vi "Andor_iXon_GetData.vi"(8 "error in":errorcluster, 11 "input cluster":T6) -> (0 "error out":errorcluster, 2 "Array 3":i32[][][](array[numeric]), 3 "array":i32[](array[numeric]))   [LabVIEW 2009]
uses:
  atmcd32d.llb/AcquisitionMode_mode typedef.ctl
  atmcd32d.llb/ReadMode_mode typedef.ctl
  atmcd32d.llb/TriggerMode_mode typedef.ctl
  atmcd32d.llb/Shutter_type typedef.ctl
  atmcd32d.llb/Shutter_mode typedef.ctl
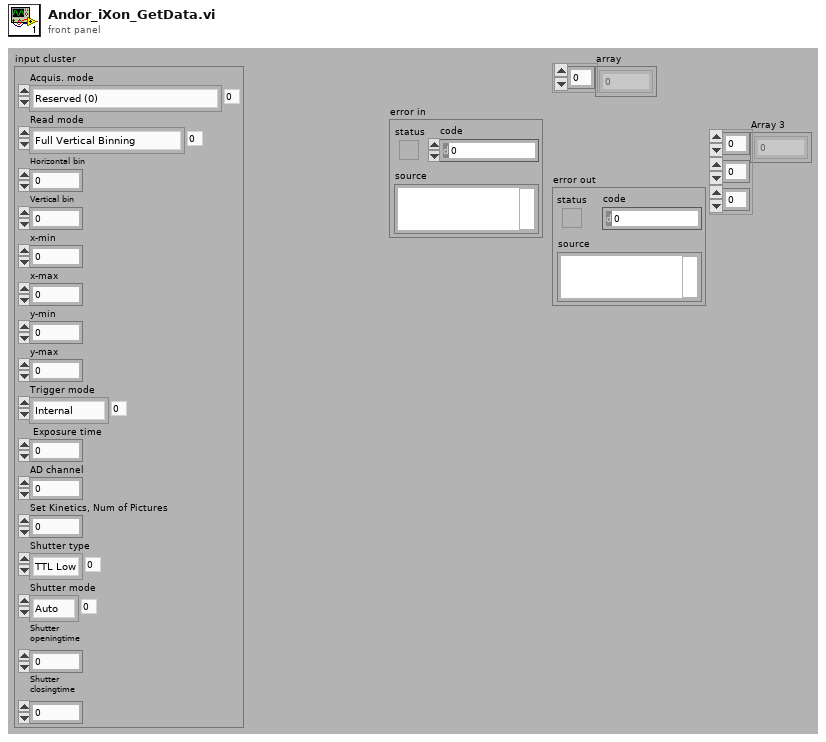
[diagram p1: front panel]
types:
  T1 = typedef "AcquisitionMode_mode typedef.ctl" = enum16{"Reserved (0)", "Single Scan", "Accumulate", "Kinetics", "Fast Kinetics", "Run Till Abort", "Reserved (6)", "Reserved (7)", "Reserved (8)", "Time Delayed Integration"}
  T2 = typedef "ReadMode_mode typedef.ctl" = enum16{"Full Vertical Binning", "Multi-Track", "Random-Track", "Single-Track", "Image"}
  T3 = typedef "TriggerMode_mode typedef.ctl" = enum16{"Internal", "External", "N/A (2)", "N/A (3)", "N/A (4)", "N/A (5)", "External Start"}
  T4 = typedef "Shutter_type typedef.ctl" = enum16{"TTL Low", "TTL High"}
  T5 = typedef "Shutter_mode typedef.ctl" = enum16{"Auto", "Open", "Close"}
  T6 = cluster{"Acquis. mode":T1, "Read mode":T2, "Horizontal bin":i32, "Vertical bin":i32, "x-min":i32, "x-max":i32, "y-min":i32, "y-max":i32, "Trigger mode":T3, " Exposure time":sgl, "AD channel":i32, "Set Kinetics, Num of Pictures":i32, "Shutter type":T4, "Shutter mode":T5, "Shutter\nopeningtime":i32, "Shutter\nclosingtime":i32}
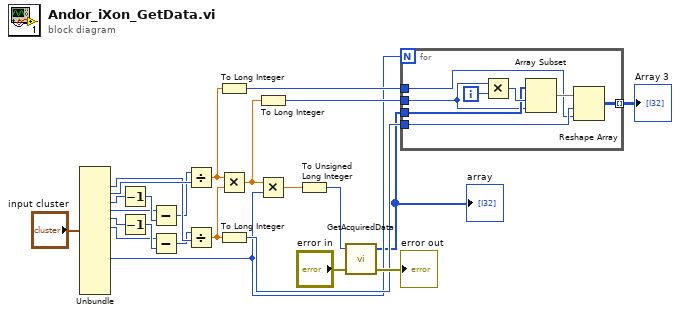
[diagram p0: block diagram]
diagram:
  n1 = Unbundle("input cluster") -> ("Horizontal bin"=w20:i32, "Vertical bin"=w21:i32, "x-min"=w11:i32, "x-max"=w4:i32, "y-min"=w3:i32, "y-max"=w5:i32, "Set Kinetics, Num of Pictures"=w14:i32)  [unwired: 9 out]
  n2 = Decrement(x=w11) -> (x-1=w10:i32)
  n3 = Decrement(x=w3) -> (x-1=w9:i32)
  n4 = Subtract(x=w4, y=w10) -> (x-y=w13:i32)
  n5 = Subtract(x=w5, y=w9) -> (x-y=w12:i32)
  n6 = Divide(x=w13, y=w21) -> (x/y=w7:dbl)
  n7 = Divide(x=w12, y=w20) -> (x/y=w8:dbl)
  n8 = To Long Integer(number=w7) -> (32bit integer=w19:i32)
  n9 = Multiply(x=w7, y=w8) -> (x*y=w15:dbl)
  n10 = To Long Integer(number=w8) -> (32bit integer=w18:i32)
  n11 = To Long Integer(number=w15) -> (32bit integer=w16:i32)
  n12 = Multiply(x=w15, y=w14) -> (x*y=w22:dbl)
  n13 = To Unsigned Long Integer(number=w22) -> (unsigned 32bit integer=w1:u32)
  n14 = call "GetAcquiredData.vi"("error in (no error)"="error in", "size"=w1) -> ("error out"=→"error out":errorcluster, "array"=w2:i32[])  [unwired: 2 out]
  "array" <- w2
  n15 = for {
    N: w14 -> [_]
    tunnel: w2 -> [w30]
    tunnel: w19 -> [w25]
    tunnel: w18 -> [w26]
    tunnel: [w29] -> w17 mode=indexing
    tunnel: w16 -> [w28]
    i -> [w27]
    n16 = Multiply(x=w28, y=w27) -> (x*y=w31:i32)
    n17 = Array Subset(array=w30, index=w31, length=w28) -> (w32:i32[])
    n18 = Reshape Array(w32, w26, w25) -> (w29:i32[][])
  }
  "Array 3" <- w17
